vi "Read ADU Packet.vi"(8 "error in":errorcluster, 10 "Network Protocol":refnum<class "Network Protocol.lvclass">, 11 "ASCII transmission data unit in":refnum<class "ASCII Data Unit.lvclass">) -> (0 "error out":errorcluster, 1 "modbus data unit":refnum<class "Modbus Data Unit.lvclass">, 2 "Network Protocol out":refnum<class "Network Protocol.lvclass">, 3 "ASCII transmission data unit out":refnum<class "ASCII Data Unit.lvclass">, 5 "PDU Valid?":bool)   [LabVIEW 2012, in "ASCII Data Unit.lvclass"]
uses:
  ASCII Data Unit.lvclass
  Modbus Data Unit/Modbus Data Unit.lvclass
  Network Protocol/Network Protocol.lvclass
  Network Protocol/Network Master/Serial/Serial Master.lvclass
  Network Protocol/Network Master/Serial/Serial Master.lvclass/Serial Master.ctl
  Network Protocol/Network Slave/Serial/Serial Slave.lvclass
  Network Protocol/Network Slave/Serial/Serial Slave.lvclass/Serial Slave.ctl
  Transmission Data Unit.lvclass/Transmission Data Unit.ctl
  Modbus Data Unit/Modbus Data Unit.lvclass/Modbus Data Unit.ctl
  ASCII Data Unit.lvclass/ASCII Data Unit.ctl
  Serial Interface/Serial acquisition states.ctl
  <vilib>/ErrorRing/Error Ring.xnode
  Transmission Data Unit.lvclass
  Serial Interface/Serial Data Unit.lvclass
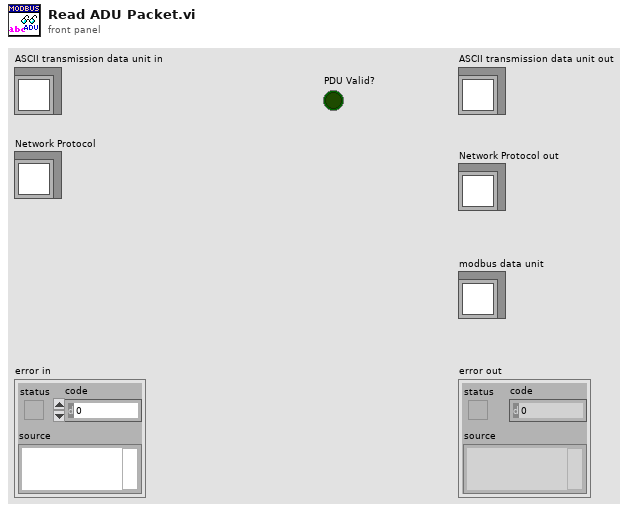
[diagram p1: front panel]
types:
  T1 = typedef "Serial Data Unit.lvclass/Serial acquisition states.ctl" = enum16{"Wait for frame", "Check for validity"}
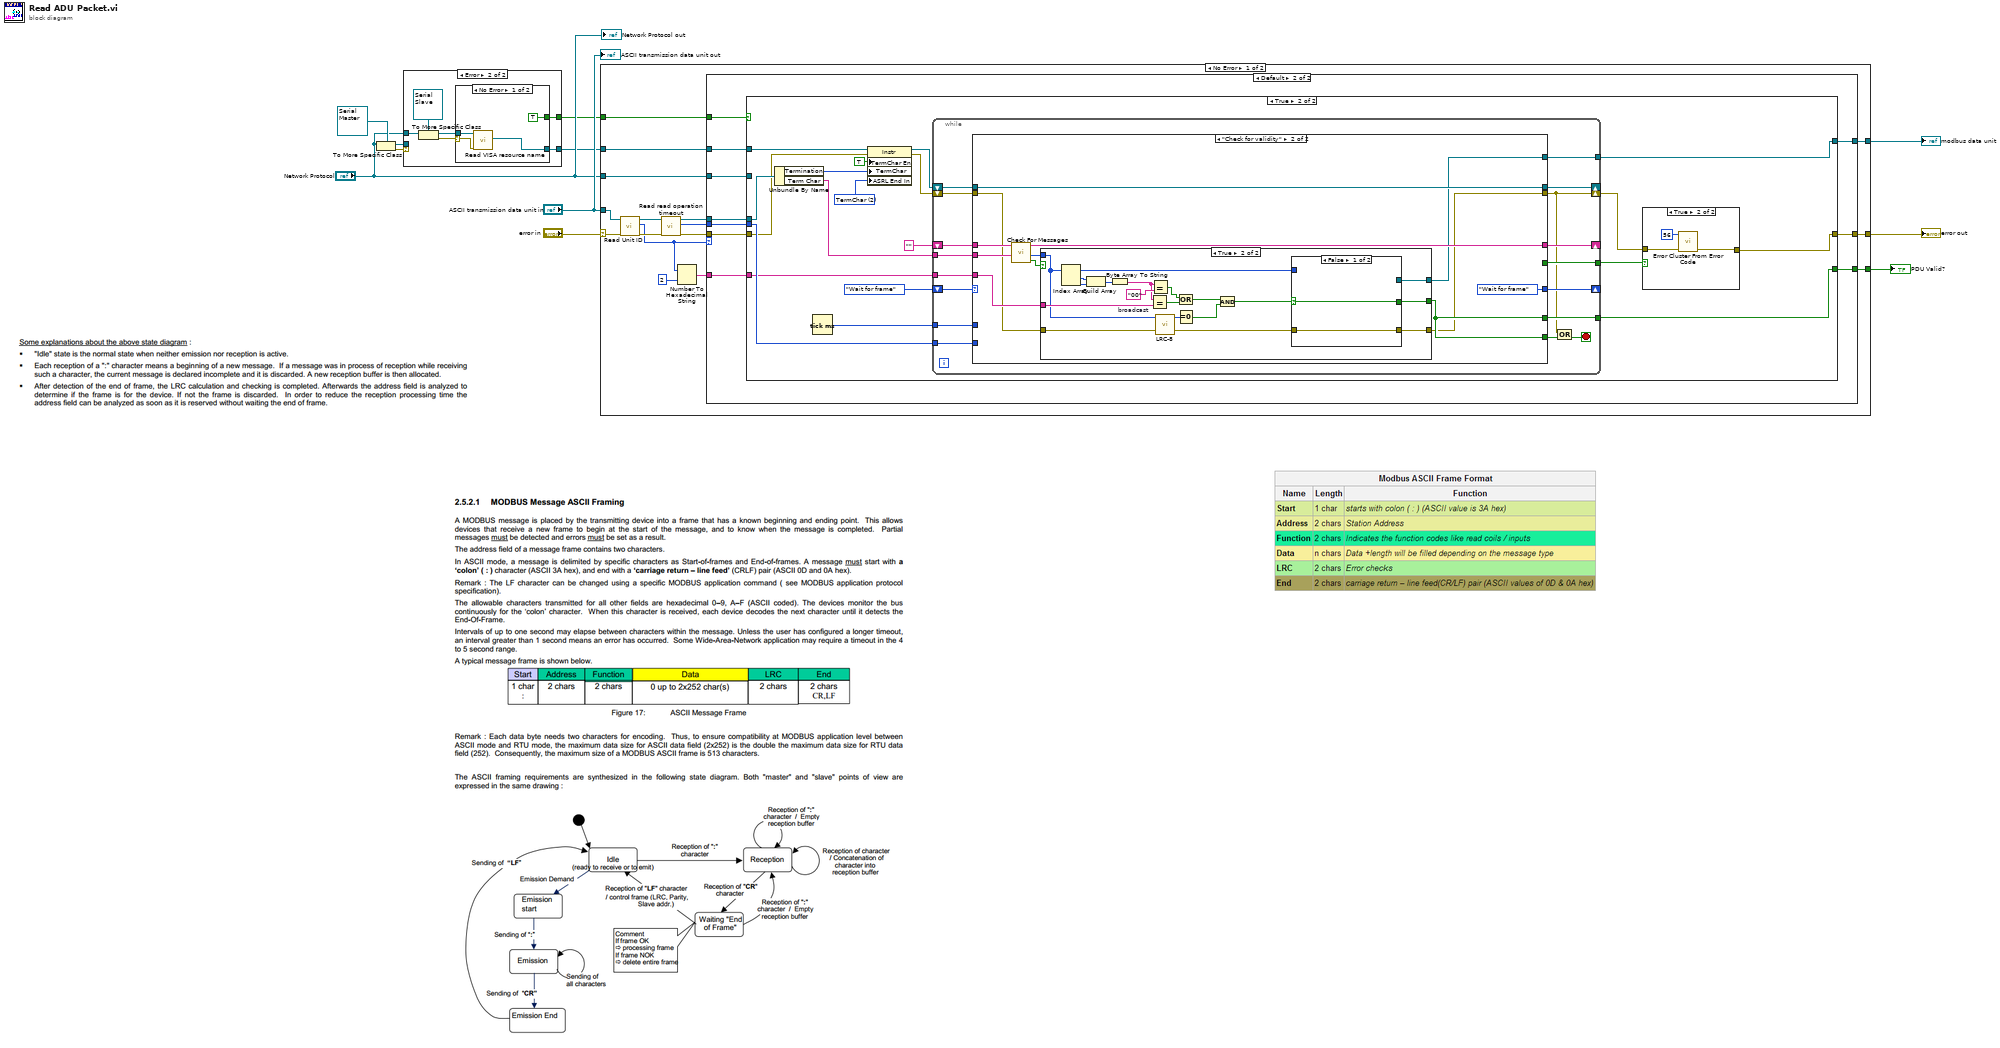
[diagram p0: block diagram]
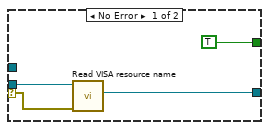
[diagram p2: hidden frame]
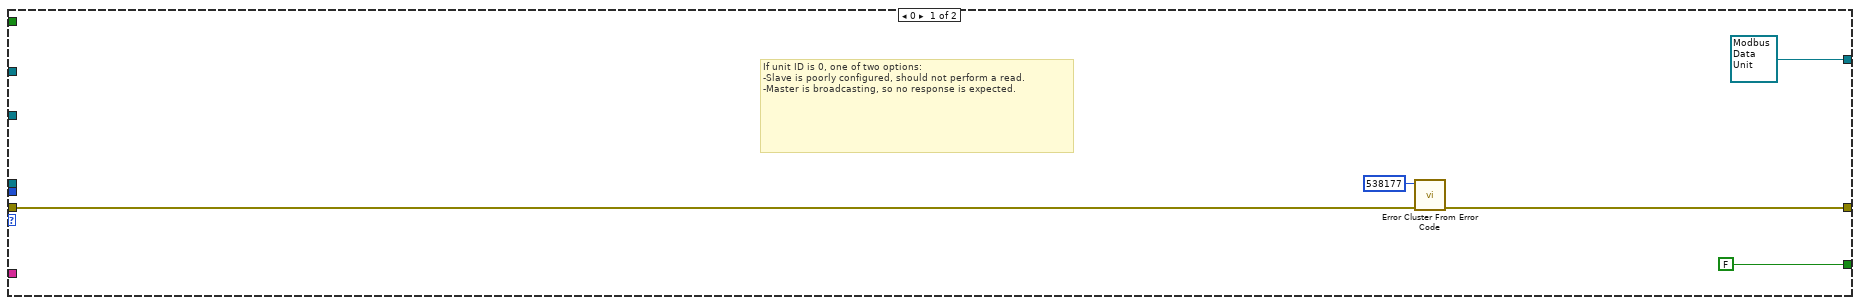
[diagram p4: hidden frame]
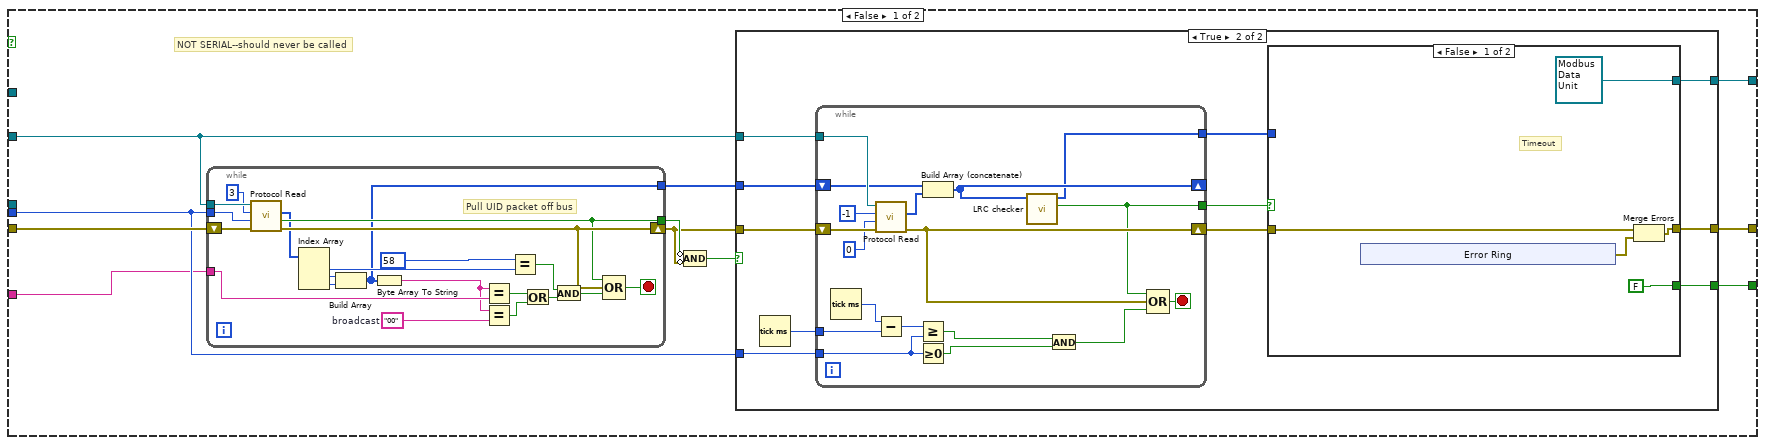
[diagram p5: hidden frame]
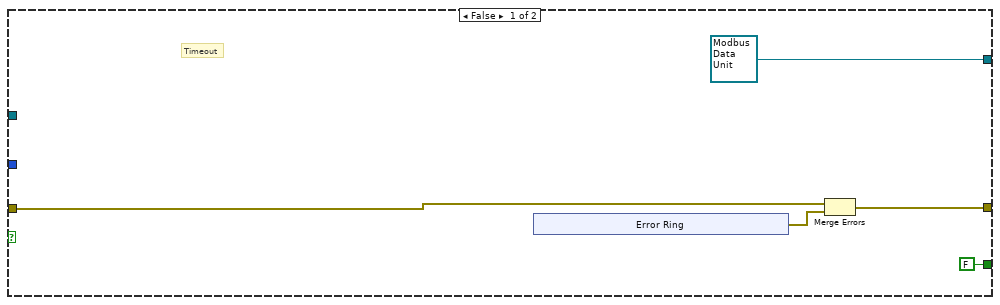
[diagram p6: hidden frame]
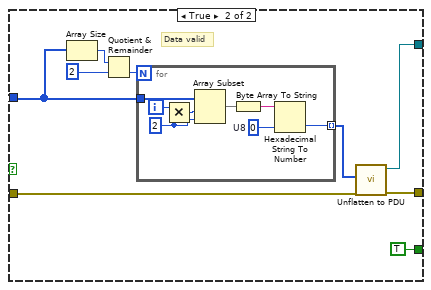
[diagram p7: hidden frame]
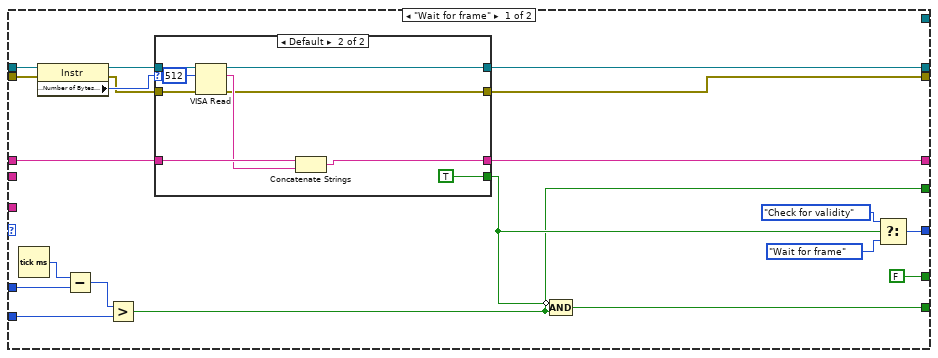
[diagram p9: hidden frame]
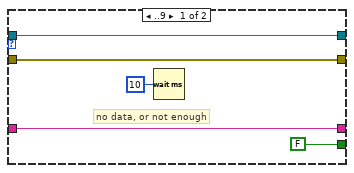
[diagram p10: hidden frame]
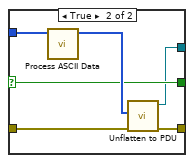
[diagram p12: hidden frame]
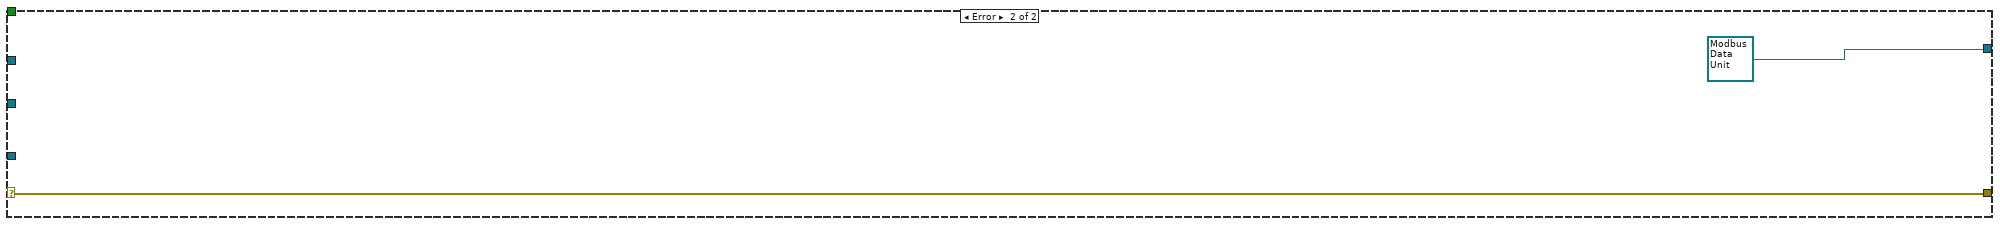
[diagram p13: hidden frame]
diagram:
  n1 = To More Specific Class(target class=refnum<class "Serial Master.lvclass"> refnum ("Serial Master"), reference="Network Protocol") -> (specific class reference=w2:refnum<class "Serial Master.lvclass">, error out=w5:errorcluster)  [unwired: 1 in]
  n2 = case shown="Error" w5 {
    selector: w5 -> [w13 _]
    tunnel: "Network Protocol" -> [_ w21]
    tunnel: [TRUE w18] -> w3
    tunnel: w2 -> [w14 _]
    tunnel: [w12 w16] -> w1
    frame No Error {
      n3 = call "Read VISA resource name.vi"("error in (no error)"=w13, "Serial Master in"=w14) -> ("VISA resource name"=w12:refnum<visa-resource-name>)  [unwired: 7 in, 2 out]
    }
    frame Error {
      n4 = To More Specific Class(target class=refnum<class "Serial Slave.lvclass"> refnum ("Serial Slave"), reference=w21) -> (specific class reference=w17:refnum<class "Serial Slave.lvclass">, error out=w19:errorcluster)  [unwired: 1 in]
      n5 = case shown="No Error" w19 {
        selector: w19 -> [w23 _]
        tunnel: [TRUE _] -> w18
        tunnel: w17 -> [w24 _]
        tunnel: [w22 _] -> w16
        frame No Error {
          n6 = call "Read VISA resource name.vi"("error in (no error)"=w23, "Serial Slave in"=w24) -> ("VISA resource name"=w22:refnum<visa-resource-name>)  [unwired: 7 in, 2 out]
        }
        frame Error {
        }
      }
    }
  }
  n7 = case shown="No Error" "error in" {
    selector: "error in" -> [w37 w267]
    tunnel: [w41 w267] -> w8
    tunnel: "ASCII transmission data unit in" -> [w27 _]
    tunnel: "Network Protocol" -> [w39 _]
    tunnel: [w40 refnum<class "Modbus Data Unit.lvclass"> refnum ("modbus data unit")] -> w9
    tunnel: [w33 _] -> w7
    tunnel: w3 -> [w32 _]
    tunnel: w1 -> [w28 _]
    frame No Error {
      n8 = call "Read Unit ID.vi"("error in"=w37, "transmission data unit in"=w27) -> ("error out"=w36:errorcluster, "unit ID"=w30:u8, "transmission data unit out"=w38:refnum<class "ASCII Data Unit.lvclass">)  [unwired: 7 in]
      n9 = call "Read read operation timeout.vi"("error in (no error)"=w36, "transmission data unit in"=w38) -> ("error out"=w35:errorcluster, "read operation timeout"=w34:i32, "transmission data unit out"=w26:refnum<class "ASCII Data Unit.lvclass">)  [unwired: 7 in]
      n10 = Number To Hexadecimal String(1:i16 2 ("width (-)"), 2:w30) -> (0:w29:string)
      n11 = case shown="Default" w30 {
        tunnel: w35 -> [w46 w52]
        tunnel: [w43 w56] -> w41
        tunnel: [refnum<class "Modbus Data Unit.lvclass"> refnum ("modbus data unit out") w55] -> w40
        tunnel: w39 -> [_ w51]
        tunnel: w34 -> [_ w54]
        tunnel: [FALSE w53] -> w33
        tunnel: w32 -> [_ w50]
        tunnel: w29 -> [_ w49]
        tunnel: w28 -> [_ w48]
        tunnel: w26 -> [_ w47]
        frame 0 {
          # "If unit ID is 0, one of two options:\n-Slave is poorly configured, should not perform a read.\n-Master is broadcasting, so no response is expected."
          n12 = call <vilib>:"Error Cluster From Error Code.vi"("error in (no error)"=w46, "error code (0)"=538177) -> ("error out"=w43:errorcluster)  [unwired: 7 in]
        }
        frame Default {
          n13 = case shown="True" w50 {
            tunnel: w52 -> [w67 w160]
            tunnel: [w63 w154] -> w56
            tunnel: [w62 w153] -> w55
            tunnel: w51 -> [w61 _]
            tunnel: w54 -> [w59 w161]
            tunnel: [w58 w159] -> w53
            tunnel: w49 -> [w57 w157]
            tunnel: w48 -> [_ w169]
            tunnel: w47 -> [_ w168]
            frame False {
              # "NOT SERIAL--should never be called"
              n14 = while {
                shift-right: [w149] -> w64
                shift-left: w67 -> [w152]
                tunnel: w59 -> [w147]
                tunnel: [w145] -> w66
                tunnel: [w137] -> w60
                tunnel: w61 -> [w151]
                tunnel: w57 -> [w138]
                stop <- w150 stop-if-true
                w132 = "00"  # broadcast
                # "Pull UID packet off bus"
                n15 = call-dynamic "Protocol Read.vi"("error in"=w152, "timeout"=w147, "bytes to read"=3, "protocol layer in"=w151) -> ("error out"=w149:errorcluster, "timed out?"=w145:bool, "data"=w144:u8[])  [unwired: 4 in, 1 out]
                n16 = Index Array(array=w144) -> (element #1=w142:u8, element #2=w140:u8, element #3=w139:u8)  [unwired: 3 in]
                n17 = Build Array(w140, w139) -> (w137:u8[])
                n18 = Byte Array To String(unsigned byte array=w137) -> (string=w133:string)
                n19 = Equal?(x=w133, y=w138) -> (x = y?=w135:bool)
                n20 = Equal?(x=w133, y=w132) -> (x = y?=w134:bool)
                n21 = Equal?(x=u8 58 ("y"), y=w142) -> (x = y?=w141:bool)
                n22 = Or(x=w135, y=w134) -> (x .or. y?=w136:bool)
                n23 = And(x=w141, y=w136) -> (x .and. y?=w146:bool)
                n24 = Compound Arithmetic op=OR(w145, w149, w146) -> (w150:bool)
              }
              n25 = Compound Arithmetic op=AND(invert w66, invert w64) -> (w65:bool)
              n26 = case shown="True" w65 {
                tunnel: w64 -> [w70 w87]
                tunnel: [w71 w79] -> w63
                tunnel: [refnum<class "Modbus Data Unit.lvclass"> refnum ("modbus data unit out") w80] -> w62
                tunnel: w61 -> [_ w83]
                tunnel: w60 -> [_ w84]
                tunnel: w59 -> [_ w85]
                tunnel: [FALSE w77] -> w58
                frame False {
                  # "Timeout"
                  n27 = xnode "Error Ring"() -> ("error out"=w72:errorcluster)
                  n28 = Merge Errors(w70, w72) -> (w71:errorcluster)
                }
                frame True {
                  n29 = Tick Count (ms)() -> (millisecond timer value=w86:u32)
                  n30 = while {
                    shift-right: [w117] -> w81
                    shift-left: w87 -> [w123]
                    tunnel: w86 -> [w131]
                    tunnel: w85 -> [w128]
                    shift-right: [w116] -> _
                    shift-left: w84 -> [w119]
                    tunnel: w83 -> [w122]
                    tunnel: [w114] -> w82
                    tunnel: [w115] -> w78
                    stop <- w125 stop-if-true
                    n31 = Tick Count (ms)() -> (millisecond timer value=w130:u32)
                    n32 = call-dynamic "Protocol Read.vi"("error in"=w123, "timeout"=0, "bytes to read"=-1, "protocol layer in"=w122) -> ("error out"=w117:errorcluster, "data"=w118:u8[])  [unwired: 4 in, 2 out]
                    n33 = Subtract(x=w130, y=w131) -> (x-y=w129:u32)
                    n34 = Greater Or Equal?(x=w129, y=w128) -> (x >= y?=w126:bool)
                    n35 = Greater Or Equal To 0?(x=w128) -> (x >= 0?=w127:bool)
                    n36 = Build Array (concatenate)(w119, w118) -> (w116:u8[])
                    n37 = call "LRC checker.vi"("Data In"=w116) -> ("Valid?"=w114:bool, "Function Data Out"=w115:u8[])  [unwired: 9 in]
                    n38 = And(x=w126, y=w127) -> (x .and. y?=w124:bool)
                    n39 = Compound Arithmetic op=OR(w114, w117, w124) -> (w125:bool)
                  }
                  n40 = case shown="False" w82 {
                    tunnel: w81 -> [w90 w103]
                    tunnel: [refnum<class "Modbus Data Unit.lvclass"> refnum ("modbus data unit") w104] -> w80
                    tunnel: [w89 w105] -> w79
                    tunnel: w78 -> [_ w98]
                    tunnel: [FALSE TRUE] -> w77
                    frame False {
                      # "Timeout"
                      n41 = xnode "Error Ring"() -> ("error out"=w91:errorcluster)
                      n42 = Merge Errors(w90, w91) -> (w89:errorcluster)
                    }
                    frame True {
                      # "Data valid"
                      n43 = Array Size(array=w98) -> (size(s)=w102:i32)
                      n44 = Quotient & Remainder(x=w102, y=2) -> (floor(x/y)=w100:i32)  [unwired: 1 out]
                      n45 = for {
                        N: w100 -> [_]
                        tunnel: w98 -> [w113]
                        tunnel: [w106] -> w99 mode=indexing
                        i -> [w112]
                        w107 = u8 0  # U8
                        w111 = 2 ("length")
                        n46 = Multiply(x=w112, y=w111) -> (x*y=w110:i32)
                        n47 = Array Subset(array=w113, index=w110, length=w111) -> (w109:u8[])
                        n48 = Byte Array To String(unsigned byte array=w109) -> (string=w108:string)
                        n49 = Hexadecimal String To Number(string=w108, default (0uL)=w107) -> (number=w106:u8)  [unwired: 2 out]
                      }
                      n50 = call "Unflatten to PDU.vi"("error in"=w103, "modbus data unit data"=w99) -> ("error out"=w105:errorcluster, "modbus data unit out"=w104:refnum<class "Modbus Data Unit.lvclass">)  [unwired: 8 in]
                    }
                  }
                }
              }
            }
            frame True {
              w170 = u16 2 items=["None", "Last Bit", "TermChar"] ("Serial Settings:End Mode for Reads")
              n51 = Unbundle By Name(w168) -> ("Termination"=w167:u8, "Term Char"=w158:string)
              n52 = Tick Count (ms)() -> (millisecond timer value=w162:u32)
              n53 = property class="Instr"(reference=w169, error in=w160, "TermChar En"=TRUE ("Message Based Settings:Termination Character Enable"), "TermChar"=w167, "ASRL End In"=w170) -> (reference out=w165:refnum<visa-resource-name>, error out=w164:errorcluster)
              n54 = while {
                shift-right: [w191] -> _
                shift-left: Serial_acquisition_states."Wait for frame" ("Serial Acquisition States") -> [w192]
                shift-right: [w176] -> w155
                shift-left: w164 -> [w189]
                shift-right: [w183] -> _
                shift-left: w165 -> [w190]
                shift-right: [w187] -> _
                shift-left: "" -> [w188]
                tunnel: w162 -> [w186]
                tunnel: w161 -> [w185]
                tunnel: [w182] -> w159
                tunnel: w158 -> [w181]
                tunnel: w157 -> [w180]
                tunnel: [w179] -> w156
                tunnel: [w178] -> w153
                stop <- w177 stop-if-true
                n55 = case shown="\"Check for validity\"" w192 {
                  tunnel: [w212 Serial_acquisition_states."Wait for frame" ("Serial Acquisition States")] -> w191
                  tunnel: w190 -> [w207 w237]
                  tunnel: w189 -> [w206 w228]
                  tunnel: w188 -> [w205 w236]
                  tunnel: [w204 w234] -> w187
                  tunnel: w186 -> [w202 _]
                  tunnel: w185 -> [w200 _]
                  tunnel: [w195 w230] -> w184
                  tunnel: [w197 w227] -> w176
                  tunnel: [w196 w237] -> w183
                  tunnel: [FALSE w230] -> w182
                  tunnel: w181 -> [_ w235]
                  tunnel: w180 -> [_ w232]
                  tunnel: [w193 _] -> w179
                  tunnel: [_ w229] -> w178
                  frame "Wait for frame" {
                    n56 = Tick Count (ms)() -> (millisecond timer value=w203:u32)
                    n57 = property class="Instr"(reference=w207, error in=w206) -> (reference out=w209:refnum<visa-resource-name>, error out=w198:errorcluster, "Serial Settings:Number of Bytes at Serial Port"=w208:u32)
                    n58 = Subtract(x=w203, y=w202) -> (x-y=w201:u32)
                    n59 = Greater?(x=w201, y=w200) -> (0:w193:bool)
                    n60 = case shown="Default" w208 {
                      tunnel: w209 -> [w213 w226]
                      tunnel: w205 -> [w216 w225]
                      tunnel: [w216 w223] -> w204
                      tunnel: [FALSE TRUE] -> w199
                      tunnel: w198 -> [w214 w221]
                      tunnel: [w214 w220] -> w197
                      tunnel: [w213 w219] -> w196
                      frame ..9 {
                        # "no data, or not enough"
                        n61 = Wait (ms)(milliseconds to wait=u32 10) -> ()  [unwired: 1 out]
                      }
                      frame Default {
                        n62 = VISA Read(VISA resource name=w226, byte count=u32 512, error in (no error)=w221) -> (VISA resource name out=w219:refnum<visa-resource-name>, read buffer=w224:string, error out=w220:errorcluster)  [unwired: 1 out]
                        n63 = Concatenate Strings(w225, w224) -> (w223:string)
                      }
                    }
                    n64 = Compound Arithmetic op=AND(invert w199, w193) -> (w195:bool)
                    n65 = Select(t=Serial_acquisition_states."Check for validity" ("Serial Acquisition States"), s=w199, f=Serial_acquisition_states."Wait for frame" ("Serial Acquisition States")) -> (s? t:f=w212:T1)
                  }
                  frame "Check for validity" {
                    n66 = call "Check For Messages.vi"("Term Char"=w235, "Input String"=w236) -> ("found?"=w231:bool, "data"=w233:u8[], "Remaining String"=w234:string)  [unwired: 7 in]
                    n67 = case shown="True" w231 {
                      selector: w231 -> [w240 _]
                      tunnel: w233 -> [_ w245]
                      tunnel: w232 -> [_ w247]
                      tunnel: w228 -> [w239 w244]
                      tunnel: [w240 w243] -> w230
                      tunnel: [_ w242] -> w229
                      tunnel: [w239 w241] -> w227
                      frame False {
                      }
                      frame True {
                        w255 = "00"  # broadcast
                        n68 = Index Array(array=w245) -> (element #1=w251:u8, element #2=w252:u8)  [unwired: 2 in]
                        n69 = Build Array(w251, w252) -> (w250:u8[])
                        n70 = Byte Array To String(unsigned byte array=w250) -> (string=w254:string)
                        n71 = Equal?(x=w254, y=w247) -> (x = y?=w248:bool)
                        n72 = Equal?(x=w254, y=w255) -> (x = y?=w253:bool)
                        n73 = call "LRC-8.vi"("data"=w245) -> ("LRC-8"=w256:u8)  [unwired: 10 in]
                        n74 = Or(x=w253, y=w248) -> (x .or. y?=w249:bool)
                        n75 = Equal To 0?(x=w256) -> (x = 0?=w257:bool)
                        n76 = Compound Arithmetic op=AND(w249, w257) -> (w246:bool)
                        n77 = case shown="False" w246 {
                          selector: w246 -> [w259 w262]
                          tunnel: w245 -> [_ w265]
                          tunnel: w244 -> [w258 w264]
                          tunnel: [w259 w262] -> w243
                          tunnel: [_ w261] -> w242
                          tunnel: [w258 w260] -> w241
                          frame False {
                          }
                          frame True {
                            n78 = call "Process ASCII Data.vi"("data"=w265) -> ("pdu"=w263:u8[])  [unwired: 10 in]
                            n79 = call "Unflatten to PDU.vi"("error in"=w264, "modbus data unit data"=w263) -> ("error out"=w260:errorcluster, "modbus data unit out"=w261:refnum<class "Modbus Data Unit.lvclass">)  [unwired: 8 in]
                          }
                        }
                      }
                    }
                  }
                }
                n80 = Or(x=w176, y=w184) -> (x .or. y?=w177:bool)
              }
              n81 = case shown="True" w156 {
                tunnel: w155 -> [w172 w175]
                tunnel: [w172 w173] -> w154
                frame False {
                }
                frame True {
                  n82 = call <vilib>:"Error Cluster From Error Code.vi"("error in (no error)"=w175, "error code (0)"=56) -> ("error out"=w173:errorcluster)  [unwired: 7 in]
                }
              }
            }
          }
        }
      }
    }
    frame Error {
    }
  }
  "modbus data unit" <- w9
  "error out" <- w8
  "PDU Valid?" <- w7
  "ASCII transmission data unit out" <- "ASCII transmission data unit in"
  "Network Protocol out" <- "Network Protocol"
